vi "fifo send AI or phase.vi"(4 "freq errors":fxp<+/-,16,1>[](array[numeric])=[0.0, 0.0, 0.0], 6 "param in":T1={"base freq (Hz)"=[0.0, 0.0, 0.0], "P gain"=[0.0, 0.0, 0.0], "I gain"=[0.0, 0.0, 0.0], "LP1 coeffs"=[0, 0, 0, 0, 0, 0, 0, 0, 0, 0, 0, 0, 0, 0, 0, 0, 0, 0], "scope on"=FALSE, "scope channel"=0, "scope signal"=0, "notch coeff"=[-1025014616, 2098093632, 165702, -1053286467, 2126356551, 167935, -1025014616, 2098093632, 165702]}, 8 "phase errrors":fxp<+/-,16,1>[](array[numeric])=[0.0, 0.0, 0.0], 9 "AI in":fxp<+/-,16,1>, 10 "AI Valid in":bool, 11 "phase":fxp<+,16,1>[](array[numeric])=[0.0, 0.0, 0.0]) -> ()   [LabVIEW 2018, in "SCTL.lvlib"]
uses:
  SCTL.lvlib
  param-sctl-pll.ctl
  <vilib>/rvi/Emulation/niFpgaEmulationIsFPGAContextNoSignature.vi
  <vilib>/rvi/Emulation/niFpgaSctlEmulationGetInTimedLoop.vi
  <vilib>/rvi/errors/niFpgaSetErrorForExecOnDevCompSimple.vi
  <vilib>/rvi/eio/common/nirviEmuReportErrorAndStop.vi
  <vilib>/rvi/DataTransferAndStorage/Container/Common/niFpgaContainerGetUniqueNameForEmu.vi
  <vilib>/rvi/FIFO/Fifo_Resource/nirvififoEmulationSetSize.vi
  <vilib>/rvi/FIFO/Fifo_Resource/nirviFifoEmulationQueueMgr.vi
  <instcachedir>/0/nirviFifoEmulationQueueMgr_E5CAEC123FF24DC58D834DCA3CDAA9B5.lvgen/nirviFifoEmulationQueueMgr_E5CAEC123FF24DC58D834DCA3CDAA9B5_000.vi
  <vilib>/rvi/FIFO/Fifo_Resource/nirvififoEmulationDetermineInputValidOut.vi
  <vilib>/rvi/FIFO/Fifo_Resource/nirvififoEmulationCreateLock.vi
  <vilib>/rvi/Emulation/niFpgaProcessEmulError.vi
  <vilib>/rvi/FIFO/Fifo_Resource/nirvififoEmulationObtainLock.vi
  <vilib>/rvi/FIFO/Fifo_Resource/nirvififoEmulationReleaseLock.vi
  <vilib>/rvi/occurrence/nirviWaitOnOccurrenceBase.vi
  <vilib>/rvi/errors/nirviReportUnexpectedCaseInternalError.vi
  <vilib>/rvi/errors/nirviReportUnexpectedCaseInternalError (U32).vi
  <vilib>/rvi/FXPMathLib/FxpInterpret/XNode/nifxpmath_Interpret.xnode
  <vilib>/rvi/DataTransferAndStorage/Container/XNode/niFpgaContainer.xnode
  <vilib>/rvi/FIFO/Fifo_Resource/nirvififoEmulationWrite.vi
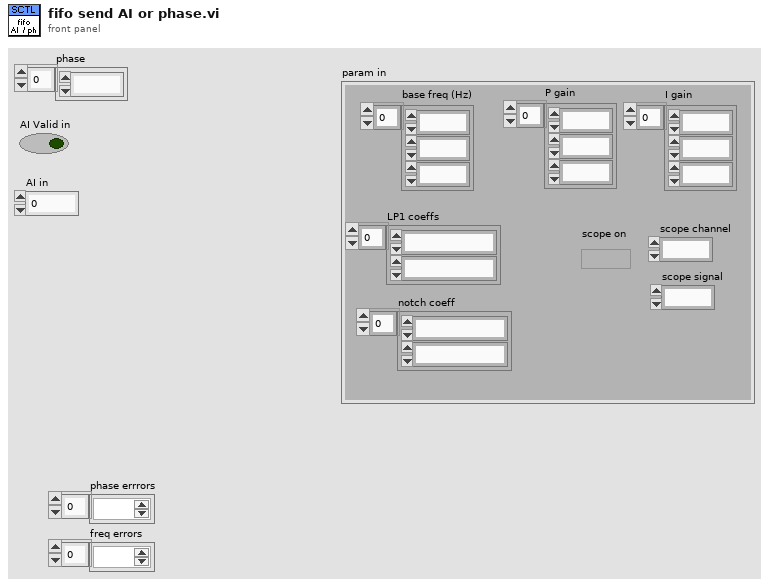
[diagram p1: front panel]
types:
  T1 = typedef "SCTL.lvlib/param-sctl-pll.ctl" = cluster{"base freq (Hz)":fxp<+,17,17>[], "P gain":fxp<+,14,14>[], "I gain":fxp<+,20,6>[], "LP1 coeffs":i32[], "scope on":bool, "scope channel":u8, "scope signal":u8, "notch coeff":i32[]}
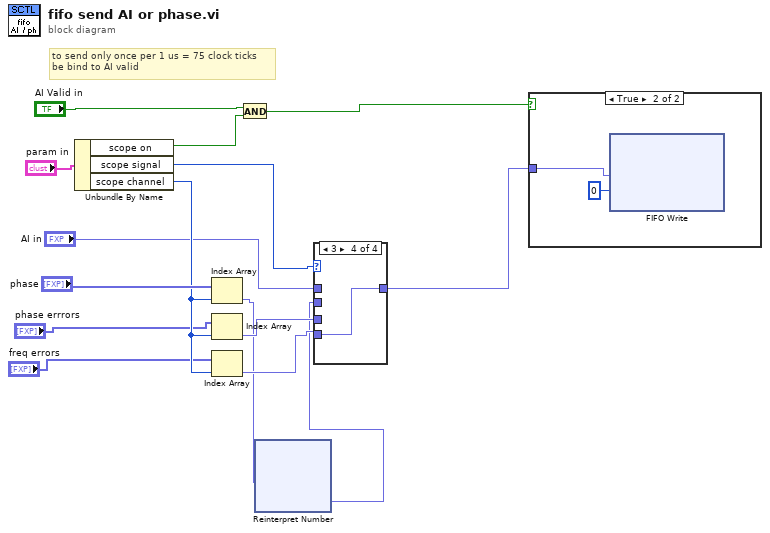
[diagram p0: block diagram]
diagram:
  # "to send only once per 1 us = 75 clock ticks\nbe bind to AI valid"
  n1 = Unbundle By Name("param in") -> ("scope on"=w14:bool, "scope signal"=w9:u8, "scope channel"=w10:u8)
  n2 = Index Array(array="phase", index=w10) -> (element=w2:fxp<+,16,1>)
  n3 = Index Array(array="phase errrors", index=w10) -> (element=w7:fxp<+/-,16,1>)
  n4 = Index Array(array="freq errors", index=w10) -> (element=w3:fxp<+/-,16,1>)
  n5 = And(x="AI Valid in", y=w14) -> (x .and. y?=w11:bool)
  n6 = xnode "Reinterpret Number"("x"=w2) -> ("y"=w1:fxp<+/-,16,1>)
  n7 = case shown="3" w9 {
    tunnel: "AI in" -> [w16 _ _ _]
    tunnel: [w16 w17 w18 w19] -> w6
    tunnel: w1 -> [_ w17 _ _]
    tunnel: w7 -> [_ _ w18 _]
    tunnel: w3 -> [_ _ _ w19]
    frame 0, Default {
    }
    frame 1 {
    }
    frame 2 {
    }
    frame 3 {
    }
  }
  n8 = case shown="True" w11 {
    tunnel: w6 -> [_ w20]
    frame False {
    }
    frame True {
      n9 = xnode ("FIFO Write")("Element"=w20, "Timeout"=0) -> ()  [unwired: 1 in, 2 out]
    }
  }
